vi "ReverseTurn.vi"(0 "Start Angle":dbl, 5 "Reversable Index":dbl) -> (7 "Target Angle":dbl)   [LabVIEW 2017]
uses:
  Robot Global Data.vi
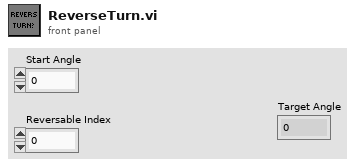
[diagram p1: front panel]
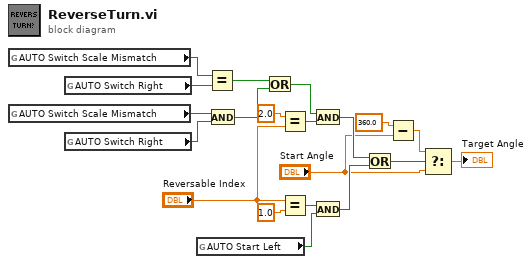
[diagram p0: block diagram]
diagram:
  n1 = global read "Robot Global Data.vi" "AUTO Switch Scale Mismatch"() -> (w10:bool)
  n2 = global read "Robot Global Data.vi" "AUTO Switch Scale Mismatch"() -> (w14:bool)
  n3 = global read "Robot Global Data.vi" "AUTO Switch Right"() -> (w11:bool)
  n4 = global read "Robot Global Data.vi" "AUTO Switch Right"() -> (w13:bool)
  n5 = global read "Robot Global Data.vi" "AUTO Start Left"() -> (w18:bool)
  n6 = Equal?(x=w10, y=w11) -> (x = y?=w9:bool)
  n7 = And(x=w14, y=w13) -> (x .and. y?=w12:bool)
  n8 = Or(x=w9, y=w12) -> (x .or. y?=w8:bool)
  n9 = Equal?(x=2.0, y="Reversable Index") -> (x = y?=w15:bool)
  n10 = Equal?(x="Reversable Index", y=1.0) -> (x = y?=w19:bool)
  n11 = And(x=w8, y=w15) -> (x .and. y?=w7:bool)
  n12 = And(x=w19, y=w18) -> (x .and. y?=w6:bool)
  n13 = Or(x=w7, y=w6) -> (x .or. y?=w5:bool)
  n14 = Subtract(x=360.0, y="Start Angle") -> (x-y=w2:dbl)
  n15 = Select(t=w2, s=w5, f="Start Angle") -> (s? t:f=→"Target Angle":dbl)
